vi "Calibrate.vi"() -> ()   [LabVIEW 2014]
panel:
  in  "Zero":bool
  in  "Motor Power":dbl(slide) scale=-1.0..1.0
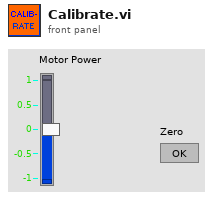
[diagram p1: front panel]
types:
  T1 = typedef "WPI_MotorControlDeviceRef.ctl" = cluster{"DeviceStatus":errorcluster, "Type":T2, "PWM":cluster{"Controller":T3, "PWM Channel":T4, "DeadBand":T5}, "CAN":cluster{"Device Number":u8, "Control Mode":T6, "Semaphore":T7, "Max Vout":dbl, "TalonSRX Control Mode":T8}, "Invert":bool, "TransformRef":T9, "InvTransformRef":T9}
  T2 = typedef "WPI_MotorControlType.ctl" = enum16{"PWM", "CAN", "CANTalonSRX"}
  T3 = typedef "FPGA_TypedefDigitalModule.ctl" = enum16{"Controller 1"}
  T4 = typedef "FPGA_DIOPWMChannel.ctl" = enum8{"PWM 0", "PWM 1", "PWM 2", "PWM 3", "PWM 4", "PWM 5", "PWM 6", "PWM 7", "PWM 8", "PWM 9", "PWM MXP 0", "PWM MXP 1", "PWM MXP 2", "PWM MXP 3", "PWM MXP 4", "PWM MXP 5", "PWM MXP 6", "PWM MXP 7", "PWM MXP 8", "PWM MXP 9", "Invalid"}
  T5 = typedef "WPI_PWMDeadband.ctl" = cluster{"Name":string, "maxPositivePwm":i32, "minPositivePwm":i32, "centerPwm":i32, "maxNegativePwm":i32, "minNegativePwm":i32, "angularRange":u16}
  T6 = typedef "WPI_CANJaguar_ControlMode.ctl" = enum8{"Percent VBus", "Current", "Speed", "Position", "Voltage"}
  T7 = typedef "Semaphore RefNum" = refnum<k1>
  T8 = typedef "WPI_CANTalonSRX_APIControlMode.ctl" = enum8{"Percent VBus", "Speed", "Position", "Slave", "Unchanged / Invalid"}
  T9 = typedef "WPI_PWMTransform_ConPane.ctl" = refnum<vi>
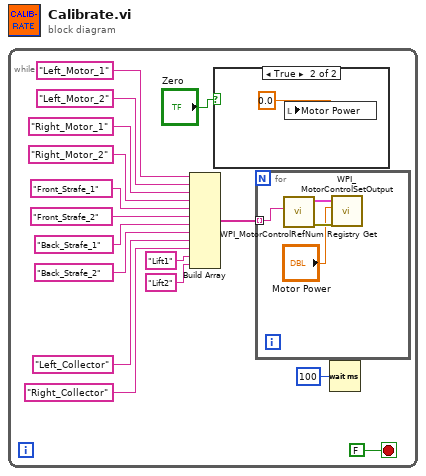
[diagram p0: block diagram]
diagram:
  n1 = while {
    stop <- FALSE stop-if-true
    n2 = Build Array("Left_Motor_1" ("refnum name"), "Left_Motor_2" ("refnum name"), "Right_Motor_1" ("refnum name"), "Right_Motor_2" ("refnum name"), "Front_Strafe_1" ("refnum name"), "Front_Strafe_2" ("refnum name"), "Back_Strafe_1" ("refnum name"), "Back_Strafe_2" ("refnum name"), "Left_Collector" ("refnum name"), "Right_Collector" ("refnum name"), "Lift1" ("refnum name"), "Lift2" ("refnum name")) -> (w3:string[])
    n3 = case shown="True" "Zero" {
      frame False {
      }
      frame True {
        n4 = local write "Motor Power"(0.0 ("Motor Power")) -> ()
      }
    }
    n5 = for {
      tunnel: w3 -> [w21] mode=indexing
      n6 = call <vilib>:"WPI_MotorControlRefNum Registry Get.vi"("refnum name"=w21) -> ("error out"=w19:errorcluster, "MotorControlDevRef"=w20:T1)  [unwired: 9 in]
      n7 = call <vilib>:"WPI_MotorControlSetOutput.vi"("error in (no error)"=w19, "Output"="Motor Power", "MotorControlDevRef"=w20) -> ()  [unwired: 6 in, 3 out]
    }
    n8 = Wait (ms)(milliseconds to wait=u32 100) -> ()  [unwired: 1 out]
  }
